vi "ASDA-A2_Initialize.vi"(8 "error in":errorcluster) -> (0 "error out":errorcluster, 3 "Buffer Data":T1)   [LabVIEW 2016]
uses:
  Data Def/ASDA-A2_Buffer Data.ctl
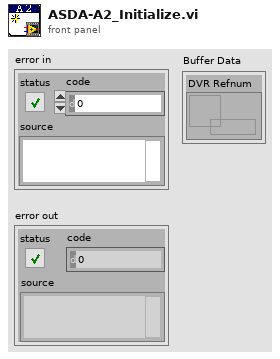
[diagram p1: front panel]
types:
  T1 = typedef "ASDA-A2_Buffer Data.ctl" = cluster{"DVR Refnum":refnum<data-value>}
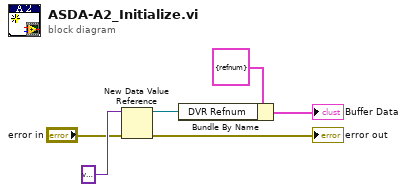
[diagram p0: block diagram]
diagram:
  n1 = New Data Value Reference(data value=variant, error in="error in") -> (data value reference=w3:refnum<data-value>, error out=→"error out":errorcluster)
  n2 = Bundle By Name(cluster=T1 {"DVR Refnum"=refnum} ("Buffer Data"), "DVR Refnum"=w3) -> (→"Buffer Data":T1)
